vi "Start Children.vi"(0 "ActorMeter in":refnum<class "ActorMeter.lvclass">, 1 "ParameterDevice.lvclass":refnum<class "ParameterDevice.lvclass">, 2 "ReadoutDevice.lvclass":refnum<class "ReadoutDevice.lvclass">, 3 "AbstractProcessor.lvclass":refnum<class "AbstractProcessor.lvclass">, 4 "AbstractCollector.lvclass":refnum<class "AbstractCollector.lvclass">, 5 "AbstractExtractor.lvclass":refnum<class "AbstractExtractor.lvclass">) -> (14 "ActorMeter out":refnum<class "ActorMeter.lvclass">)   [LabVIEW 2014, in "ActorMeter.lvclass"]
uses:
  ActorMeter.lvclass
  Hardware/ReadoutDevice/ReadoutDevice.lvclass
  Hardware/ParameterDevice/ParameterDevice.lvclass
  Collector/AbstractCollector/AbstractCollector.lvclass
  Processor/AbstractProcessor/AbstractProcessor.lvclass
  Extractor/AbstractExtractor/AbstractExtractor.lvclass
  <vilib>/ActorFramework/Actor/Actor.lvclass/Actor.ctl
  <vilib>/ActorFramework/Message Enqueuer/Message Enqueuer.lvclass/Message Enqueuer.ctl
  ActorMeter.lvclass/ActorMeter.ctl
  <vilib>/ActorFramework/Message Enqueuer/Init from Existing Queue.vi
  <vilib>/ActorFramework/Message Enqueuer/Message Enqueuer.lvclass
  <vilib>/ActorFramework/Actor/Actor.lvclass
  Interfaces/Pipelined Actor/Pipelined Actor.lvclass
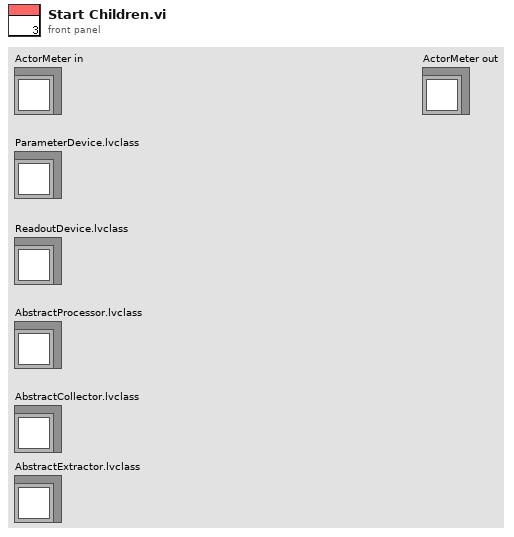
[diagram p1: front panel]
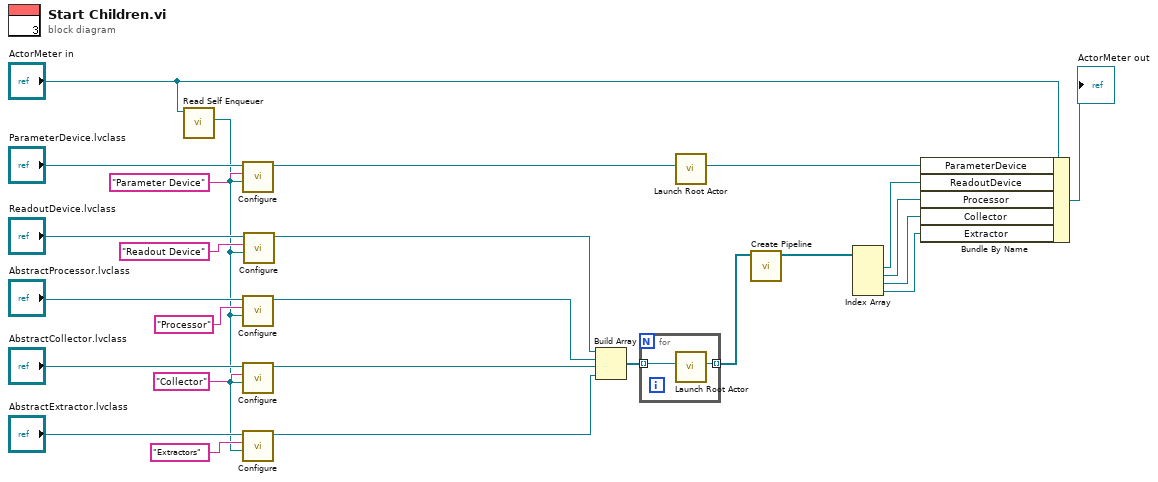
[diagram p0: block diagram]
diagram:
  n1 = call <vilib>:"Read Self Enqueuer.vi"("Actor"="ActorMeter in") -> ("Self Enqueuer"=w1:refnum<class "Message Enqueuer.lvclass">)  [unwired: 10 in]
  n2 = call-dynamic "Configure.vi"("ActorMeter Enqueuer"=w1, "Name"="Parameter Device", "Viewable Actor in"="ParameterDevice.lvclass") -> ("Viewable Actor out"=w16:refnum<class "ParameterDevice.lvclass">)  [unwired: 7 in, 1 out]
  n3 = call-dynamic "Configure.vi"("ActorMeter Enqueuer"=w1, "Name"="Processor", "Viewable Actor in"="AbstractProcessor.lvclass") -> ("Viewable Actor out"=w12:refnum<class "AbstractProcessor.lvclass">)  [unwired: 7 in, 1 out]
  n4 = call-dynamic "Configure.vi"("ActorMeter Enqueuer"=w1, "Name"="Collector", "Viewable Actor in"="AbstractCollector.lvclass") -> ("Viewable Actor out"=w10:refnum<class "AbstractCollector.lvclass">)  [unwired: 7 in, 1 out]
  n5 = call-dynamic "Configure.vi"("ActorMeter Enqueuer"=w1, "Name"="Extractors", "Viewable Actor in"="AbstractExtractor.lvclass") -> ("Viewable Actor out"=w8:refnum<class "AbstractExtractor.lvclass">)  [unwired: 7 in, 1 out]
  n6 = call-dynamic "Configure.vi"("ActorMeter Enqueuer"=w1, "Name"="Readout Device", "Viewable Actor in"="ReadoutDevice.lvclass") -> ("Viewable Actor out"=w14:refnum<class "ReadoutDevice.lvclass">)  [unwired: 7 in, 1 out]
  n7 = Build Array(w14, w12, w10, w8) -> (w24:refnum<class "Pipelined Actor.lvclass">[])
  n8 = for {
    tunnel: w24 -> [w28] mode=indexing
    tunnel: [w27] -> w26 mode=indexing
    n9 = call <vilib>:"Launch Root Actor.vi"("Actor"=w28) -> ("Actor's Enqueuer"=w27:refnum<class "Message Enqueuer.lvclass">)  [unwired: 9 in, 1 out]
  }
  n10 = call <vilib>:"Launch Root Actor.vi"("Actor"=w16) -> ("Actor's Enqueuer"=w22:refnum<class "Message Enqueuer.lvclass">)  [unwired: 9 in, 1 out]
  n11 = call "Create Pipeline.vi"("Array in"=w26) -> ("Array out"=w25:refnum<class "Message Enqueuer.lvclass">[])  [unwired: 8 in, 2 out]
  n12 = Index Array(array=w25) -> (element #1=w18:refnum<class "Message Enqueuer.lvclass">, element #2=w19:refnum<class "Message Enqueuer.lvclass">, element #3=w20:refnum<class "Message Enqueuer.lvclass">, element #4=w21:refnum<class "Message Enqueuer.lvclass">)  [unwired: 4 in]
  n13 = Bundle By Name(cluster="ActorMeter in", "ParameterDevice"=w22, "ReadoutDevice"=w18, "Processor"=w19, "Collector"=w20, "Extractor"=w21) -> (→"ActorMeter out":refnum<class "ActorMeter.lvclass">)
